vi "Scan_from_string.vi"() -> ()   [LabVIEW 2019]
panel:
  in  "Input data":string="As of 10 May 2020 The Number of patients recovered from corona \nvirus in India is Maharashtra 3800, Gujrat is 2091 and Tamil Nadu is 1959."
  out "Tamil Nadu":i32=1959
  out "Gujrat":i32=2091
  out "Maharashtra":i32=3800
  out "year":i32=2020
  out "month":string="May"
  out "day":i32=10
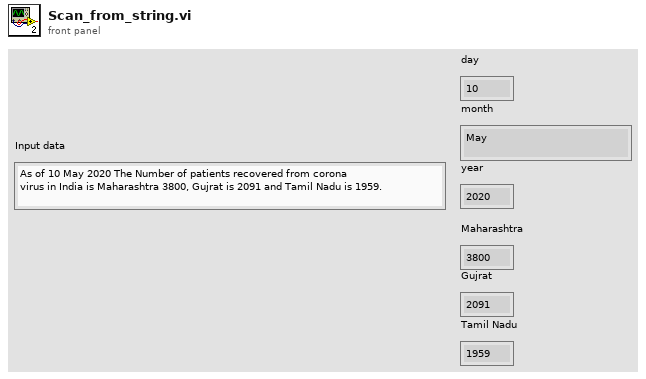
[diagram p1: front panel]
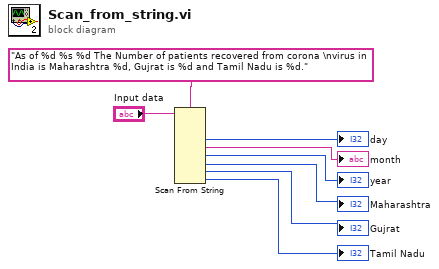
[diagram p0: block diagram]
diagram:
  n1 = Scan From String(format string="As of %d %s %d The Number of patients recovered from corona \nvirus in India is Maharashtra %d, Gujrat is %d and Tamil Nadu is %d.", input string="Input data") -> (output 1=→"day":i32, output 2=→"month":string, output 3=→"year":i32, output 4=→"Maharashtra":i32, output 5=→"Gujrat":i32, output 6=→"Tamil Nadu":i32)  [unwired: 8 in, 3 out]
